vi "Wait for Plugin Started.vi"(8 "error in (no error)":errorcluster, 9 "Timeout (ms)":i32, 11 "pCOMM Ref 2":T1) -> (0 "error out":errorcluster, 3 "Generic Plugin out":refnum<class "Generic Plugin.lvclass">)   [LabVIEW 2011, in "Generic Plugin.lvclass"]
uses:
  Generic Plugin.lvclass
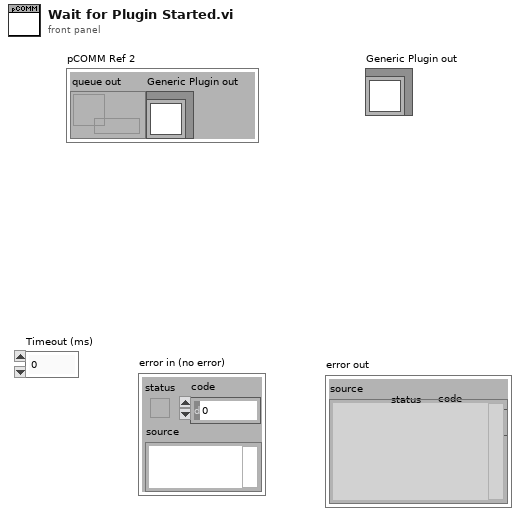
[diagram p1: front panel]
types:
  T1 = cluster{"queue out":refnum<queue>, "Generic Plugin out":refnum<class "Generic Plugin.lvclass">}
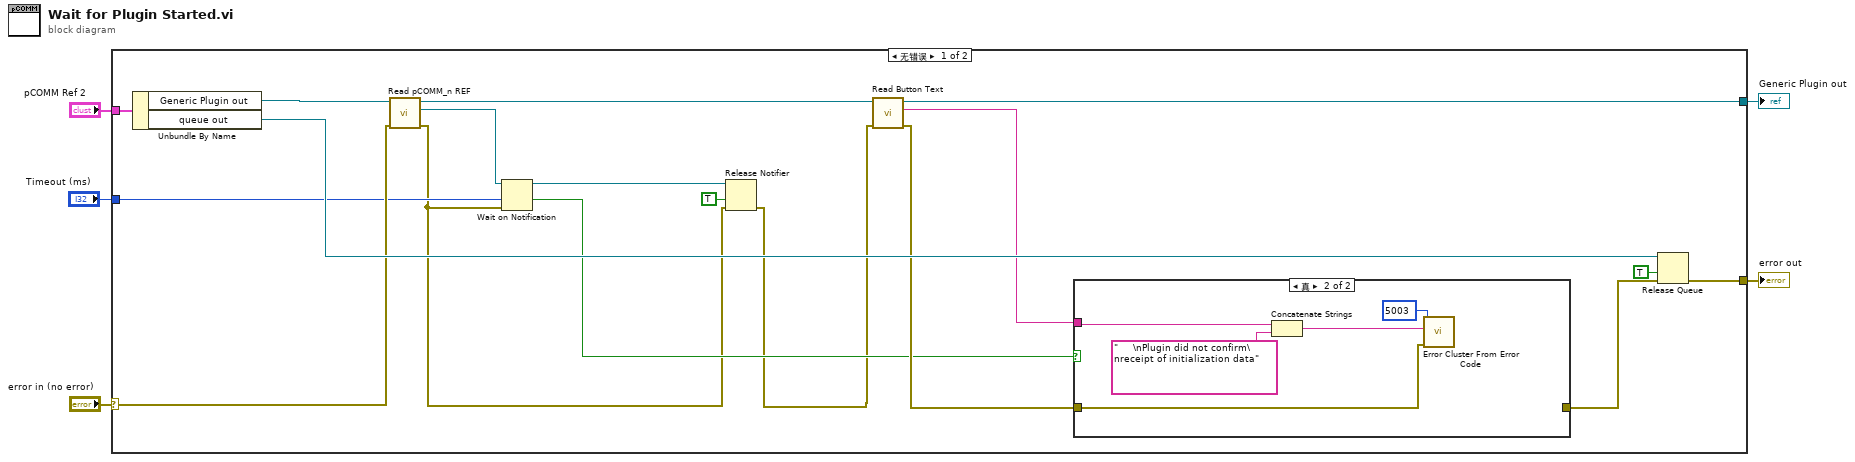
[diagram p0: block diagram]
diagram:
  n1 = case shown="无错误" "error in (no error)" {
    selector: "error in (no error)" -> [w16 w30]
    tunnel: [w22 w30] -> w5
    tunnel: "pCOMM Ref 2" -> [w23 _]
    tunnel: [w17 _] -> w2
    tunnel: "Timeout (ms)" -> [w12 _]
    frame No Error {
      n2 = Unbundle By Name(w23) -> ("Generic Plugin out"=w15:refnum<class "Generic Plugin.lvclass">, "queue out"=w21:refnum<queue>)
      n3 = call "Read pCOMM_n REF.vi"("error in (no error)"=w16, "Generic Plugin in"=w15) -> ("error out"=w7:errorcluster, "pCOMM_n REF"=w13:refnum<notifier>, "Generic Plugin out"=w14:refnum<class "Generic Plugin.lvclass">)  [unwired: 7 in]
      n4 = Wait on Notification(notifier=w13, timeout in ms (-1)=w12, error in (no error)=w7) -> (notifier out=w10:refnum<notifier>, timed out?=w11:bool)  [unwired: 1 in, 2 out]
      n5 = Release Notifier(notifier=w10, force destroy? (F)=TRUE, error in (no error)=w7) -> (error out=w9:errorcluster)  [unwired: 2 out]
      n6 = call-dynamic "Read Button Text.vi"("error in (no error)"=w9, "Generic Plugin in"=w14) -> ("error out"=w18:errorcluster, "Button Text"=w20:string, "Generic Plugin out"=w17:refnum<class "Generic Plugin.lvclass">)  [unwired: 7 in]
      n7 = case shown="真" w11 {
        tunnel: [w24 _] -> w19
        tunnel: w20 -> [_ w27]
        tunnel: w18 -> [w24 w26]
        frame False {
        }
        frame True {
          n8 = Concatenate Strings(w27, "     \nPlugin did not confirm\nreceipt of initialization data" ("error message (\"\")")) -> (w25:string)
          n9 = call <vilib>:"Error Cluster From Error Code.vi"("error in (no error)"=w26, "error message (\"\")"=w25, "error code (0)"=5003) -> ()  [unwired: 6 in, 1 out]
        }
      }
      n10 = Release Queue(queue=w21, force destroy? (F)=TRUE, error in (no error)=w19) -> (error out=w22:errorcluster)  [unwired: 2 out]
    }
    frame Error {
    }
  }
  "error out" <- w5
  "Generic Plugin out" <- w2
